vi "Timestamp to String.vi"(9 "UTC? (F)":bool, 10 "Timestamp (now)":timestamp, 11 "DateTimeFormatter in":refnum<class "DateTimeFormatter.lvclass">) -> (1 "Not a Timestamp?":bool, 2 "DateTime String":string, 3 "DateTimeFormatter out":refnum<class "DateTimeFormatter.lvclass">)   [LabVIEW 2018, in "DateTimeFormatter.lvclass"]
uses:
  DateTimeFormatter.lvclass
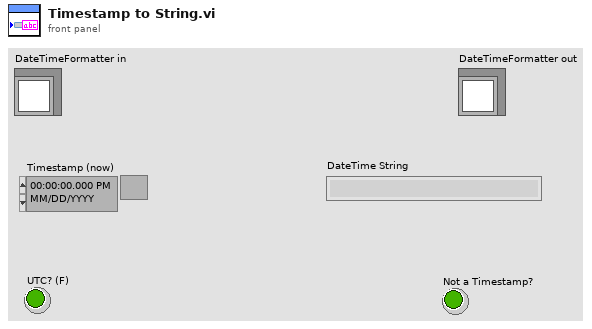
[diagram p1: front panel]
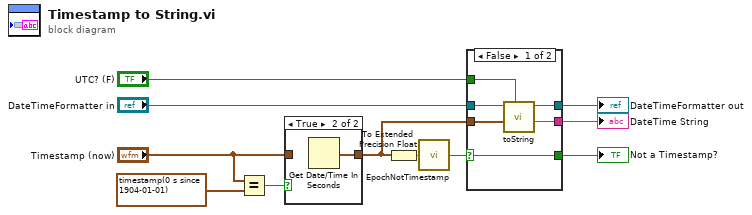
[diagram p0: block diagram]
diagram:
  n1 = Equal?(x="Timestamp (now)", y=timestamp(0 s since 1904-01-01) ("x")) -> (x = y?=w8:bool)
  n2 = case shown="True" w8 {
    tunnel: [w12 w13] -> w6
    tunnel: "Timestamp (now)" -> [w12 _]
    frame False {
    }
    frame True {
      n3 = Get Date/Time In Seconds() -> (seconds since 1Jan1904=w13:timestamp)
    }
  }
  n4 = To Extended Precision Float(1:w6) -> (0:w7:ext)
  n5 = call "EpochNotTimestamp.vi"("Epoch Time"=w7) -> ("Not a Timestamp?"=w3:bool)  [unwired: 8 in]
  n6 = case shown="False" w3 {
    selector: w3 -> [w14 w21]
    tunnel: "DateTimeFormatter in" -> [w19 w20]
    tunnel: [w18 w20] -> w10
    tunnel: w6 -> [w17 _]
    tunnel: [w16 _] -> w5
    tunnel: "UTC? (F)" -> [w15 _]
    tunnel: [w14 w21] -> w2
    frame False {
      n7 = call-dynamic "toString.vi"("UTC? (F)"=w15, "Timestamp (now)"=w17, "DateTimeFormatter in"=w19) -> ("DateTime String"=w16:string, "DateTimeFormatter out"=w18:refnum<class "DateTimeFormatter.lvclass">)  [unwired: 7 in]
    }
    frame True {
    }
  }
  "DateTimeFormatter out" <- w10
  "DateTime String" <- w5
  "Not a Timestamp?" <- w2
